vi "IR dat reader (2).vi"() -> ()   [LabVIEW 2012]
uses:
  <vilib>/Utility/file.llb/Read From Spreadsheet File (I64).vi
panel:
  in  "refresh":bool
  in  "Stop":bool
  in  "Listbox":i32(listbox)
  out "Waveform Graph":i64[][](graph)
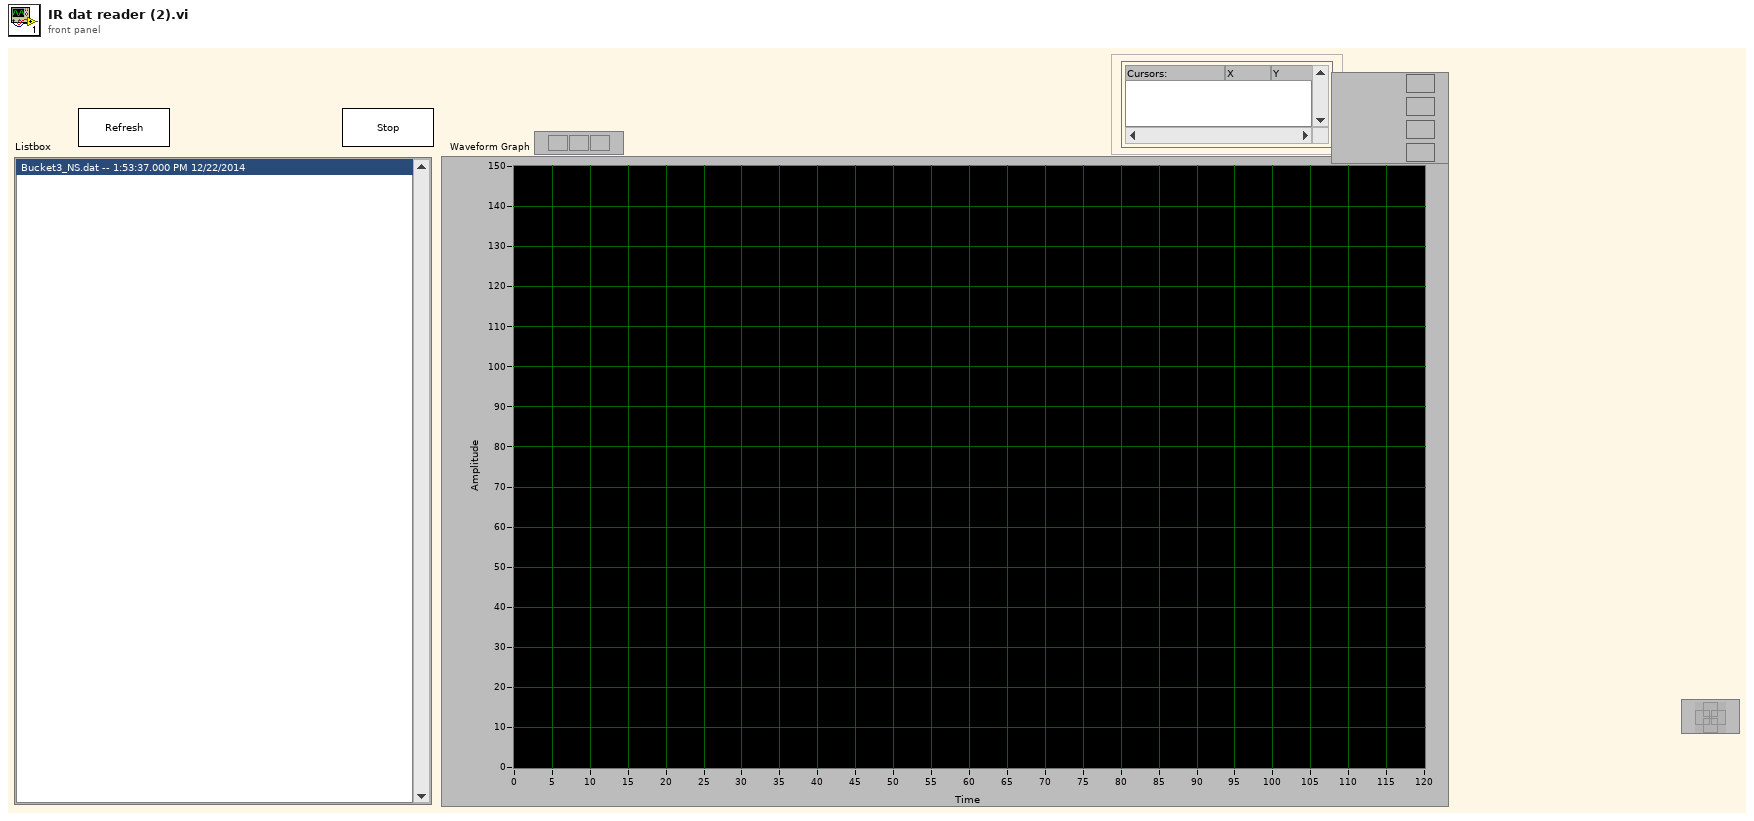
[diagram p1: front panel]
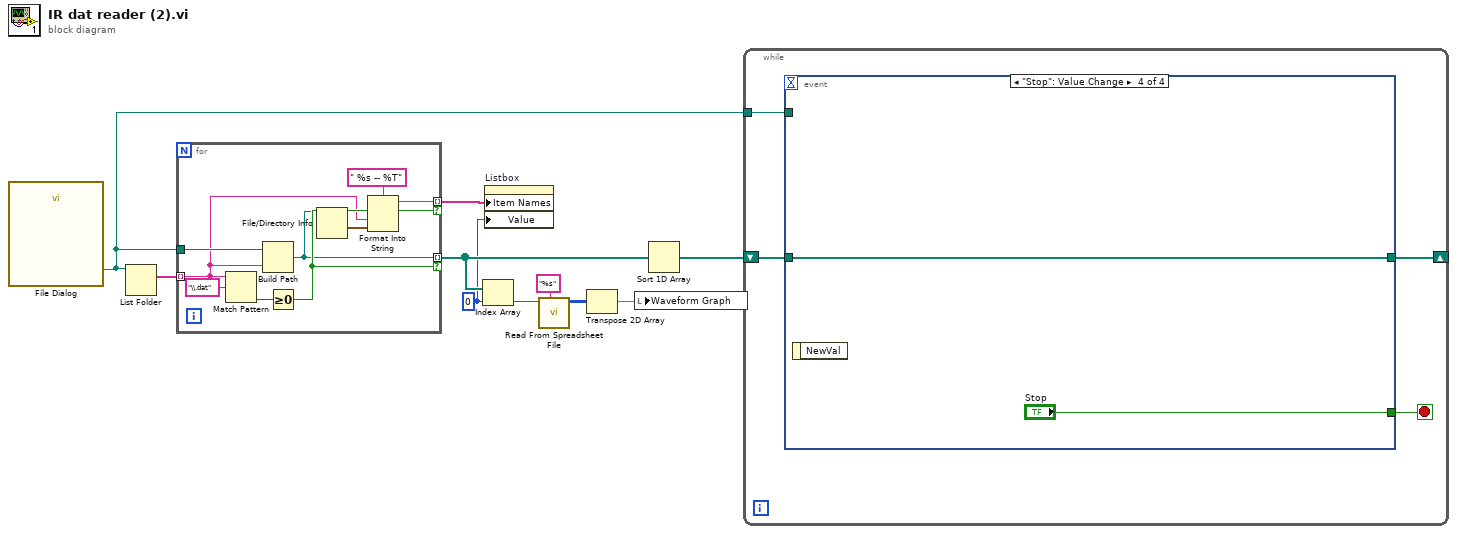
[diagram p0: block diagram]
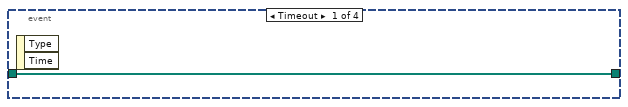
[diagram p2: hidden frame]
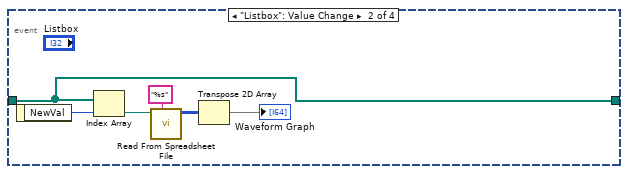
[diagram p3: hidden frame]
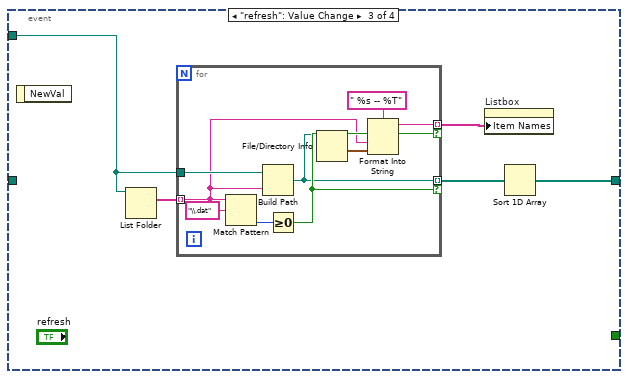
[diagram p4: hidden frame]
diagram:
  w3 = 0 ("index")
  n1 = call "File Dialog"() -> ("selected path"=w2:path)  [unwired: 12 in, 3 out]
  n2 = List Folder(path=w2) -> (filenames=w10:string[])  [unwired: 3 in, 3 out]
  n3 = for {
    tunnel: w10 -> [w13] mode=indexing
    tunnel: w2 -> [w17]
    tunnel: [w11] -> w9 mode=indexing if=w16
    tunnel: [w15] -> w8 mode=indexing if=w16
    n4 = Match Pattern(string=w13, regular expression="\\.dat") -> (offset past match=w18:i32)  [unwired: 1 in, 3 out]
    n5 = Build Path(base path=w17, name or relative path=w13) -> (appended path=w15:path)
    n6 = Greater Or Equal To 0?(x=w18) -> (x >= 0?=w16:bool)
    n7 = File/Directory Info(path=w15) -> (last mod=w14:timestamp)  [unwired: 1 in, 6 out]
    n8 = Format Into String(format string=" %s -- %T", w13, w14) -> (resulting string=w11:string)  [unwired: 2 in, 1 out]
  }
  n9 = Index Array(array=w8, index=w3) -> (element=w5:path)
  n10 = property on="Listbox" class="LstBox (strict)"("Item Names"=w9, "Value"=w3) -> ()  [unwired: 2 in, 2 out]
  n11 = call-poly <vilib>:"Read From Spreadsheet File.vi"("format (%d)"="%s", "file path (dialog if empty)"=w5) -> ("all rows"=w6:i64[][])  [unwired: 5 in, 4 out]
  n12 = Transpose 2D Array(2D array=w6) -> (transposed array=w4:i64[][])
  n13 = local write "Waveform Graph"(w4) -> ()
  n14 = Sort 1D Array(array=w8) -> (sorted array=w1:path[])
  n15 = while {
    shift-right: [w21] -> _
    shift-left: w1 -> [w23]
    tunnel: w2 -> [w20]
    stop <- w22 stop-if-true
    n16 = event shown="[3] \"Stop\": Value Change" {
      selector: _ -> [_ _ _ _]
      dyn-events: _ -> [_ _ _ _]
      timeout: _ -> [_ _ _ _]
      tunnel: w23 -> [w24 w27 _ w45]
      tunnel: [_ _ _ "Stop"] -> w22
      tunnel: [w24 w27 w31 w45] -> w21
      tunnel: w20 -> [_ _ w33 _]
      event Timeout {
        n17 = event-data() -> ()  [unwired: 1 in, 2 out]
      }
      event "Listbox": Value Change {
        n18 = event-data() -> ("NewVal"=w26:i32)  [unwired: 1 in]
        n19 = Index Array(array=w27, index=w26) -> (element=w25:path)
        n20 = call-poly <vilib>:"Read From Spreadsheet File.vi"("format (%d)"="%s", "file path (dialog if empty)"=w25) -> ("all rows"=w30:i64[][])  [unwired: 5 in, 4 out]
        n21 = Transpose 2D Array(2D array=w30) -> (transposed array=→"Waveform Graph":i64[][])
      }
      event "refresh": Value Change {
        n22 = event-data() -> ()  [unwired: 1 in, 1 out]
        n23 = List Folder(path=w33) -> (filenames=w34:string[])  [unwired: 3 in, 3 out]
        n24 = for {
          tunnel: w34 -> [w38] mode=indexing
          tunnel: w33 -> [w42]
          tunnel: [w36] -> w35 mode=indexing if=w41
          tunnel: [w40] -> w32 mode=indexing if=w41
          n25 = Match Pattern(string=w38, regular expression="\\.dat") -> (offset past match=w43:i32)  [unwired: 1 in, 3 out]
          n26 = Build Path(base path=w42, name or relative path=w38) -> (appended path=w40:path)
          n27 = Greater Or Equal To 0?(x=w43) -> (x >= 0?=w41:bool)
          n28 = File/Directory Info(path=w40) -> (last mod=w39:timestamp)  [unwired: 1 in, 6 out]
          n29 = Format Into String(format string=" %s -- %T", w38, w39) -> (resulting string=w36:string)  [unwired: 2 in, 1 out]
        }
        n30 = property on="Listbox" class="LstBox (strict)"("Item Names"=w35) -> ()  [unwired: 2 in, 2 out]
        n31 = Sort 1D Array(array=w32) -> (sorted array=w31:path[])
      }
      event "Stop": Value Change {
        n32 = event-data() -> ()  [unwired: 1 in, 1 out]
      }
    }
  }
